vi "Get CCD Status.vi"(8 "error in (no error)":errorcluster, 11 "RxTx in":refnum<class "RxTx.lvclass">) -> (0 "error out":errorcluster, 3 "RxTx out":refnum<class "RxTx.lvclass">)   [LabVIEW 2018, in "RxTx.lvclass"]
uses:
  RxTx.lvclass
  RxTx.lvclass/RxTx.ctl
  Interface/Interface.lvclass
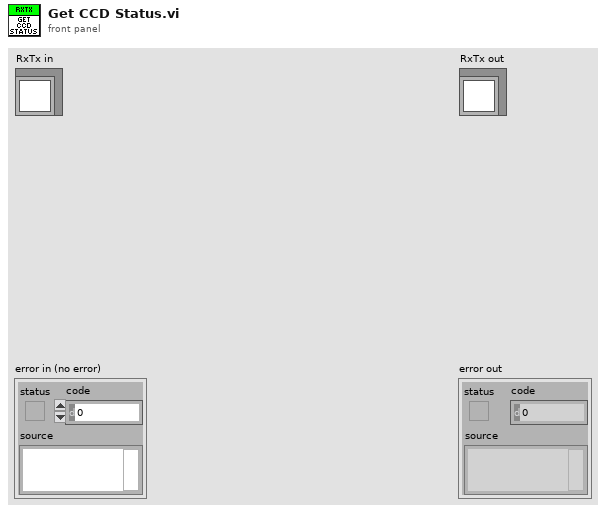
[diagram p1: front panel]
types:
  T1 = cluster{"CUBE_EXPOSURE_TIME":sgl, "CUBES_DONE":u16, "LAST_IMAGE_NAME":string, "DISK_SPACE":u16, "FRAMES_DONE":u16, "CCD_STATUS":string, "CURRENT_TEMPERATURE":i16, "TEMPERATURE_STATUS":string, "FRAME_EXPOSURE_TIME":sgl, "CCD_POWER_STATUS":bool, "SERIAL_NUMBER":u16, "ACQUIRING":bool}
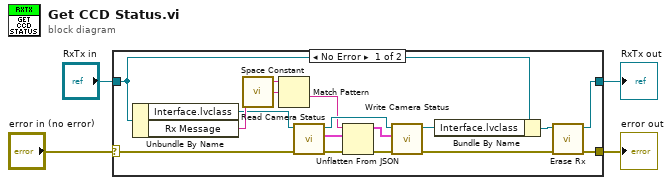
[diagram p0: block diagram]
diagram:
  n1 = case shown="No Error" "error in (no error)" {
    selector: "error in (no error)" -> [w14 w22]
    tunnel: [w11 w22] -> w2
    tunnel: [w12 w21] -> w1
    tunnel: "RxTx in" -> [w17 w21]
    frame No Error {
      n2 = Unbundle By Name(w17) -> ("Interface.lvclass"=w15:refnum<class "Interface.lvclass">, "Rx Message"=w18:string)
      n3 = call <vilib>:"Space Constant.vi"() -> ("String"=w20:string)
      n4 = Match Pattern(string=w18, regular expression=w20) -> (after substring=w9:string)  [unwired: 1 in, 3 out]
      n5 = call "Read Camera Status.vi"("error in (no error)"=w14, "Interface in"=w15) -> ("error out"=w6:errorcluster, "Camera Status"=w8:T1, "Interface out"=w16:refnum<class "Interface.lvclass">)  [unwired: 7 in]
      n6 = Unflatten From JSON(JSON string=w9, type and defaults=w8, error in (no error)=w6) -> (value=w5:T1, error out=w7:errorcluster)  [unwired: 4 in]
      n7 = call "Write Camera Status.vi"("error in (no error)"=w7, "Camera Status"=w5, "Interface in"=w16) -> ("error out"=w10:errorcluster, "Interface out"=w19:refnum<class "Interface.lvclass">)  [unwired: 7 in]
      n8 = Bundle By Name(cluster=w17, "Interface.lvclass"=w19) -> (w13:refnum<class "RxTx.lvclass">)
      n9 = call "Erase Rx.vi"("error in (no error)"=w10, "RxTx in"=w13) -> ("error out"=w11:errorcluster, "RxTx out"=w12:refnum<class "RxTx.lvclass">)  [unwired: 8 in]
    }
    frame Error {
    }
  }
  "error out" <- w2
  "RxTx out" <- w1
